vi "Check and Create Folder.vi"(8 "error in (no error)":errorcluster, 11 "Path In":path) -> (0 "error out":errorcluster, 2 "file or folder exists?":bool, 3 "Path Out":path)   [LabVIEW 2019]
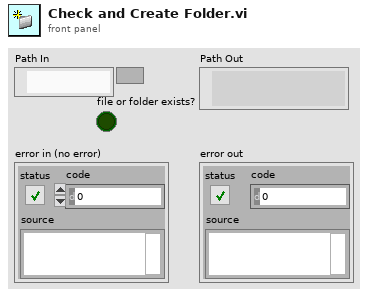
[diagram p1: front panel]
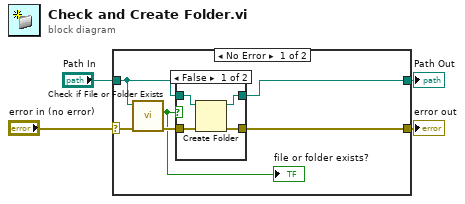
[diagram p0: block diagram]
diagram:
  n1 = case shown="No Error" "error in (no error)" {
    selector: "error in (no error)" -> [w6 w17]
    tunnel: [w10 w18] -> w4
    tunnel: [w9 w17] -> w3
    tunnel: "Path In" -> [w8 w18]
    frame No Error {
      n2 = call <vilib>:"Check if File or Folder Exists.vi"("error in (no error)"=w6, "path"=w8) -> ("error out"=w7:errorcluster, "file or folder exists?"=w5:bool)  [unwired: 7 in, 1 out]
      "file or folder exists?" <- w5
      n3 = case shown="False" w5 {
        tunnel: w7 -> [w14 w16]
        tunnel: w8 -> [w13 w15]
        tunnel: [w12 w16] -> w9
        tunnel: [w11 w15] -> w10
        frame False {
          n4 = Create Folder(path (use dialog)=w13, error in=w14) -> (created path=w11:path, error out=w12:errorcluster)  [unwired: 1 in, 1 out]
        }
        frame True {
        }
      }
    }
    frame Error {
    }
  }
  "Path Out" <- w4
  "error out" <- w3
